vi "System Message.vi"(7 "Sys. Msg. Source":T1, 8 "error in (no error)":errorcluster, 9 "Payload":variant, 10 "Identifier":string) -> (0 "error out":errorcluster)   [LabVIEW 2020, in "DBModule.lvlib"]
doc: "Broadcast a system generic message.\n____\nHAMPEL SOFTWARE ENGINEERING v2.6.0 (2023-12-19 10:54)"
uses:
  DBModule.lvlib
  Libraries/hse-libraries/Source/hse-dqmh/Controls/System Message Source.ctl
  System Message Argument--cluster.ctl
  Libraries/hse-libraries/Source/hse-dqmh/hse-dqmh.lvlib
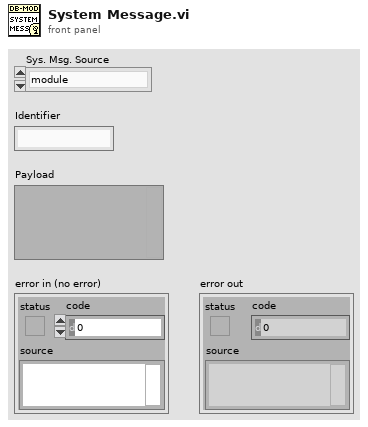
[diagram p1: front panel]
types:
  T1 = typedef "hse-dqmh.lvlib/System Message Source.ctl" = enum16{"module", "application", "network"}
  T2 = typedef "DBModule.lvlib/System Message Argument--cluster.ctl" = cluster{"Identifier":string, "Payload":variant, "Sys. Msg. Source":T1, "Sys. Msg. Origin":string}
  T3 = typedef "DBModule.lvlib/Broadcast Events--cluster.ctl" = cluster{"Module Did Init":refnum<user-event>, "Status Updated":refnum<user-event>, "Error Reported":refnum<user-event>, "Module Did Stop":refnum<user-event>, "Update Module Execution Status":refnum<user-event>, "System Message":refnum<user-event>}
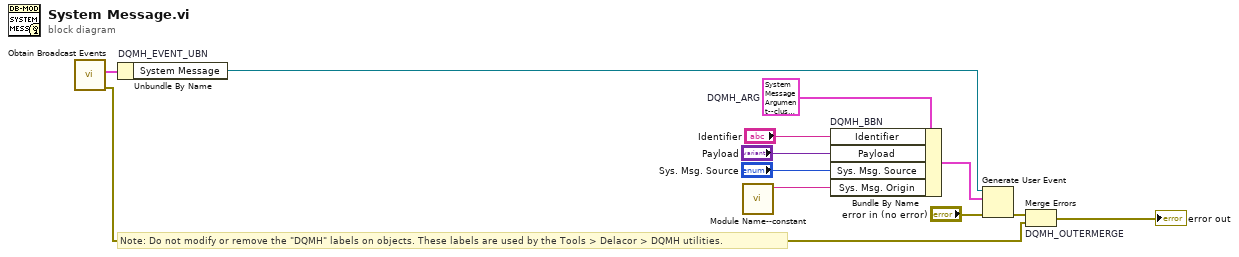
[diagram p0: block diagram]
diagram:
  w7 = T2 {"Identifier"="", "Payload"=variant, "Sys. Msg. Source"=enum."module", "Sys. Msg. Origin"=""}  # DQMH_ARG
  # "Note: Do not modify or remove the \"DQMH\" labels on objects. These labels are used by the Tools > Delacor > DQMH utilities."
  n1 = call "Obtain Broadcast Events.vi"() -> ("error out"=w3:errorcluster, "DBModule Broadcast Events"=w2:T3)  [unwired: 10 in]
  n2 = Unbundle By Name "DQMH_EVENT_UBN"(w2) -> ("System Message"=w9:refnum<user-event>)
  n3 = call "Module Name--constant.vi"() -> ("Module Name"=w1:string)  [unwired: 11 in]
  n4 = Bundle By Name "DQMH_BBN"(cluster=w7, "Identifier"="Identifier", "Payload"="Payload", "Sys. Msg. Source"="Sys. Msg. Source", "Sys. Msg. Origin"=w1) -> (w10:T2)
  n5 = Generate User Event(user event=w9, event data cluster=w10, error in="error in (no error)") -> (error out=w8:errorcluster)  [unwired: 1 in, 1 out]
  n6 = Merge Errors "DQMH_OUTERMERGE"(w8, w3) -> (→"error out":errorcluster)
